vi "Load Instrument Classes_New.vi"(8 "error in (no error)":errorcluster, 11 "C.E.":refnum<class "Control Experiment.lvclass">) -> (0 "error out":errorcluster, 3 "Control Experiment":refnum<class "Control Experiment.lvclass">)   [LabVIEW 2019, in "Control Experiment.lvclass"]
uses:
  Control Experiment.lvclass
  <userlib>/LevyLab/Instrument Framework/SMOs/Instrument/Instrument.lvclass
  Control Experiment.lvclass/Control Experiment.ctl
  <userlib>/LevyLab/Lockin-Multichannel/Instrument.Lockin/Instrument.Lockin.lvclass
  C:/Program Files (x86)/National Instruments/LabVIEW 2019/user.lib/LevyLab/Instrument Framework/SMOs/Instrument/Instrument.lvclass
  Typedefs/Instrument Types--combo.ctl
  <userlib>/LevyLab/Instrument Framework/SMOs/Instrument/Instrument.lvclass/Instrument.ctl
  <userlib>/LevyLab/Krohn Hite 7008/Instrument.KH7008.lvclass
  <vilib>/Utility/Data Type/NI_Data Type.lvlib
panel:
  out "String":string
  in  "Lockin":cluster{"Lockin Address":string} caption="Instruments"
  in  "Instruments (addresses)":T1 caption="Instruments"
  in  "KH Addresses":refnum<visa-resource-name>[](array[refnum])=["COM20", "COM14"] caption="Krohn Hite"
  in  "OK":bool
  in  "Instruments (classes)":T2 {"Capacitance Bridge" items=["", "AH2500A"]; "Level" items=["", "Instrument.TC.CF", "Instrument.TC.MNK", "Instrument.Oxford1820", "instrument.PPMS", "instrument.PPMS1", "instrument.PPMS2", "instrument.PPMS3"]; "Rotator" items=["", "Instrument.TC.CF", "Instrument.TC.MNK", "Instrument.Oxford1820", "instrument.PPMS", "instrument.PPMS1", "instrument.PPMS2", "instrument.PPMS3"]; "Magnet" items=["", "Instrument.TC.CF", "Instrument.TC.MNK", "Instrument.Oxford1820", "instrument.PPMS", "instrument.PPMS1", "instrument.PPMS2", "instrument.PPMS3"]; "Temperature" items=["", "Instrument.TC.CF", "Instrument.TC.MNK", "Instrument.Oxford1820", "instrument.PPMS", "instrument.PPMS1", "instrument.PPMS2", "instrument.PPMS3"]}
  # "1. Choose or confirm instrument classes"
  # "2. Choose or confirm addresses"
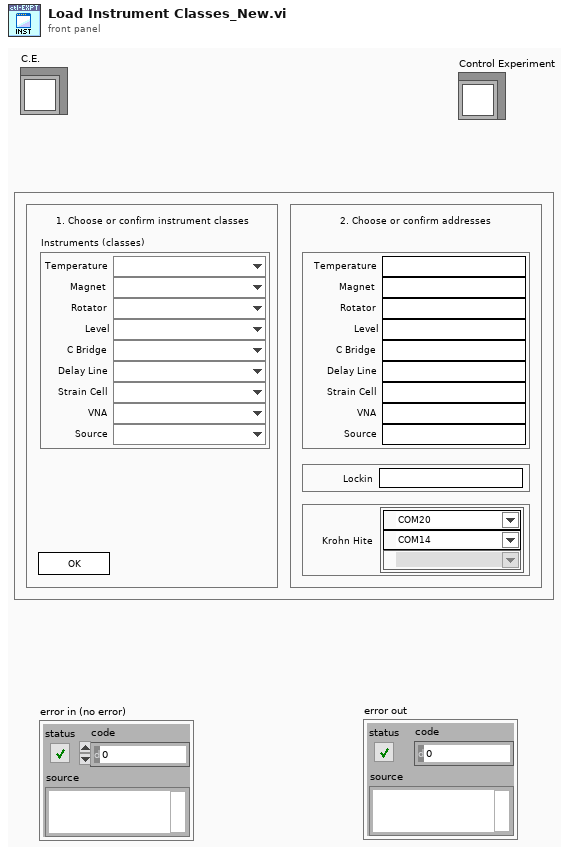
[diagram p1: front panel]
types:
  T1 = cluster{"Temperature":string, "Magnet":string, "Rotator":string, "Level":string, "Capacitance Bridge":string, "Delay Line":string, "Strain Cell":string, "VNA":string, "Source":string}
  T2 = cluster{"Temperature":u16, "Magnet":u16, "Rotator":u16, "Level":u16, "Capacitance Bridge":u16, "Delay Line":u16, "Strain Cell":u16, "VNA":u16, "Source":u16}
  T3 = enum32{"Invalid", "Standard", "Closed", "Hidden", "Minimized", "Maximized"}
  T4 = enum32{"invalid app kind", "Development System", "Run Time System", "Student Edition", "Embedded LabVIEW", "Evaluation", "Custom"}
  T5 = typedef "Control Experiment.lvclass/Instrument Types--combo.ctl" = string
  T6 = cluster{"Core":cluster{"Current VI Reference":refnum<vi>, "Close Panel on Exit?":bool}, "C.E.":refnum<class "Control Experiment.lvclass">, "Instruments":refnum<vi>, "Addresses":refnum<vi>, "Rings":refnum<vi>[], "Installed Instruments":refnum<class "Instrument.lvclass">[], "Cast Instruments":refnum<class "Instrument.lvclass">[]}
  T7 = cluster{"Current VI Reference":refnum<vi>, "Close Panel on Exit?":bool}
  T8 = enum32{"Bad", "Idle", "Run top level", "Running"}
  T9 = cluster{"class path":path, "Address":string, "Type":T5}[]
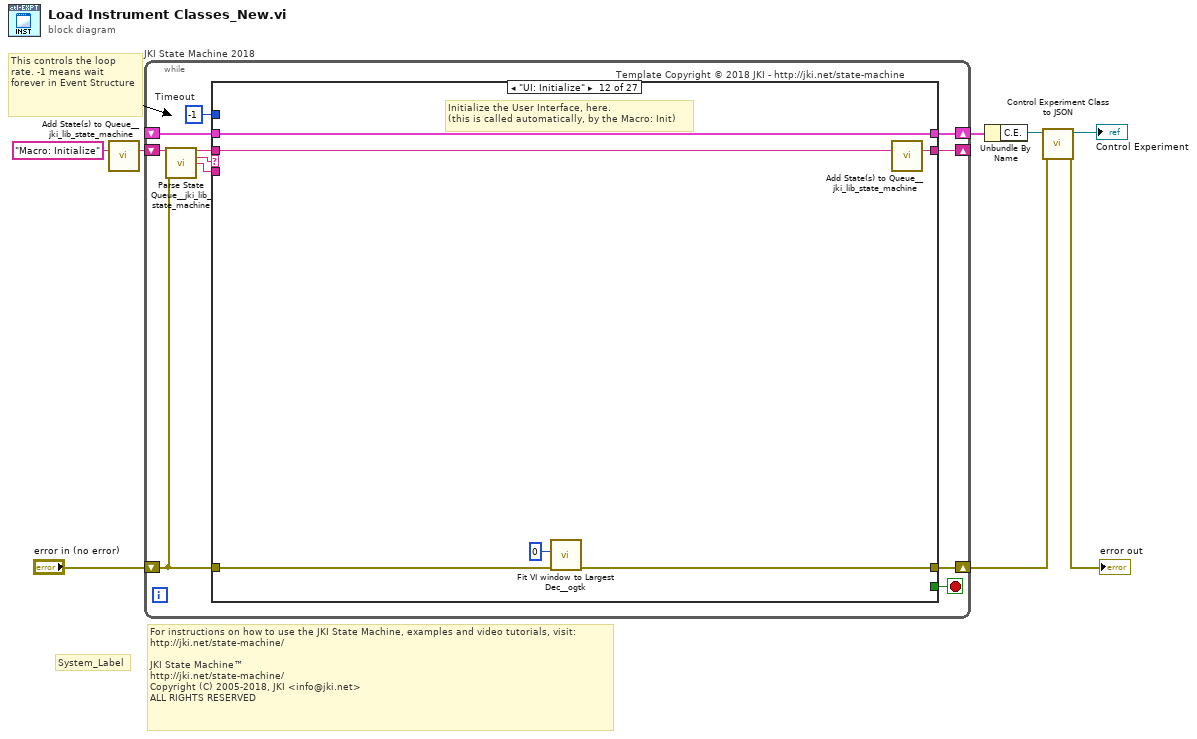
[diagram p0: block diagram]
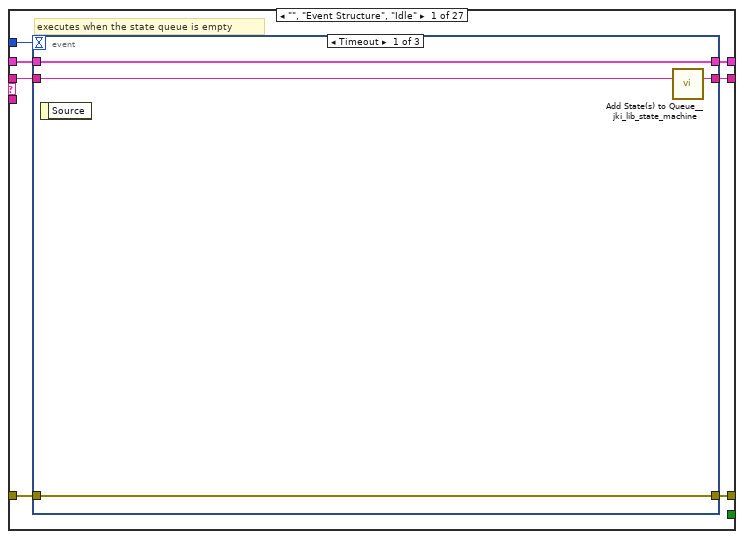
[diagram p2: hidden frame]
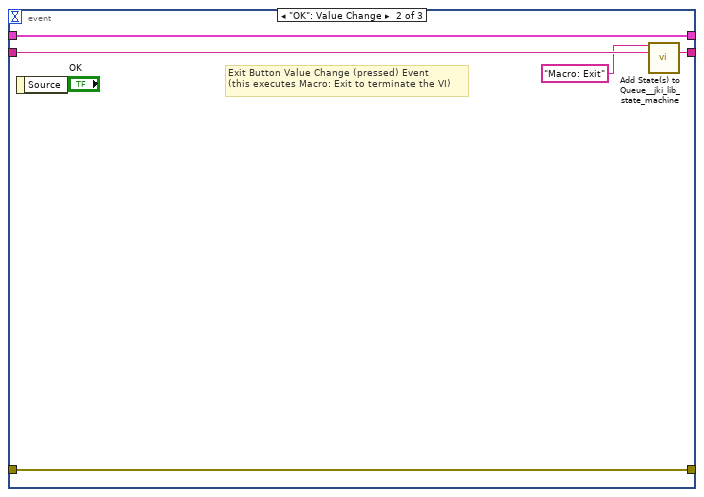
[diagram p3: hidden frame]
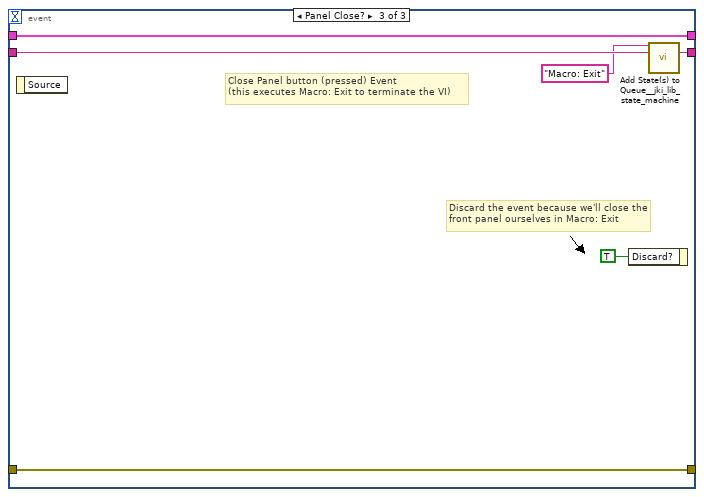
[diagram p4: hidden frame]
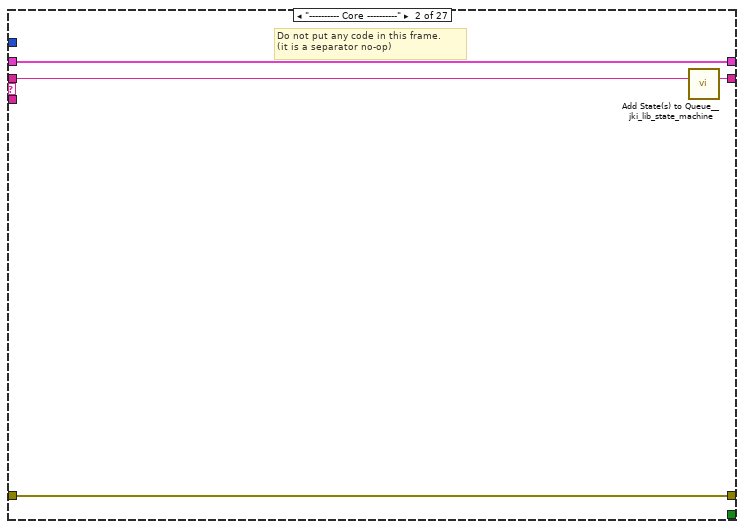
[diagram p5: hidden frame]
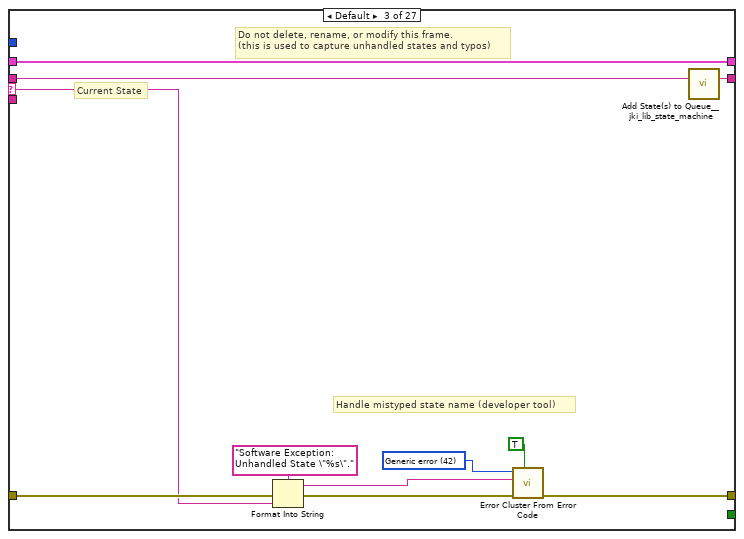
[diagram p6: hidden frame]
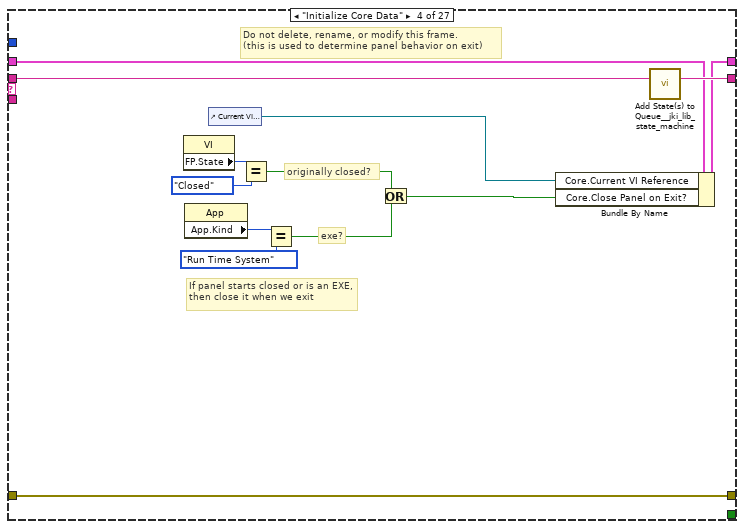
[diagram p7: hidden frame]
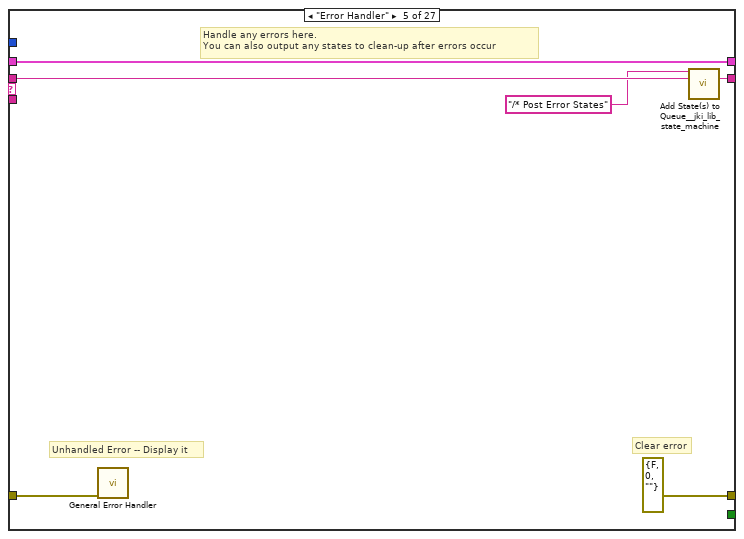
[diagram p8: hidden frame]
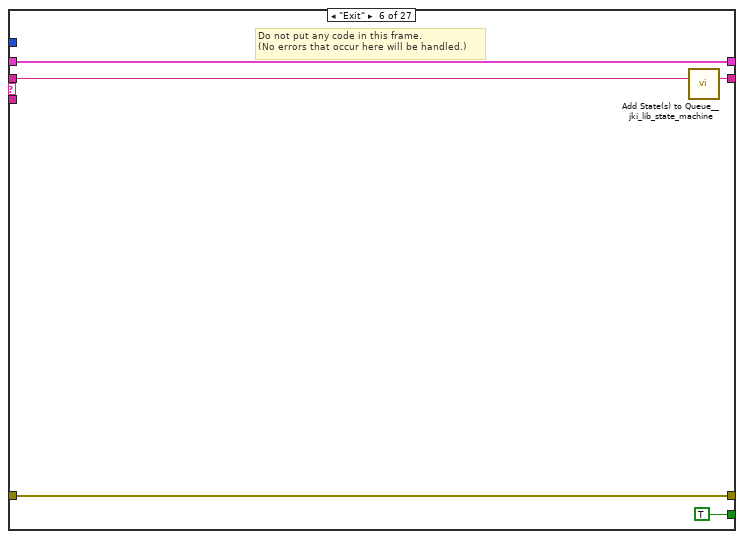
[diagram p9: hidden frame]
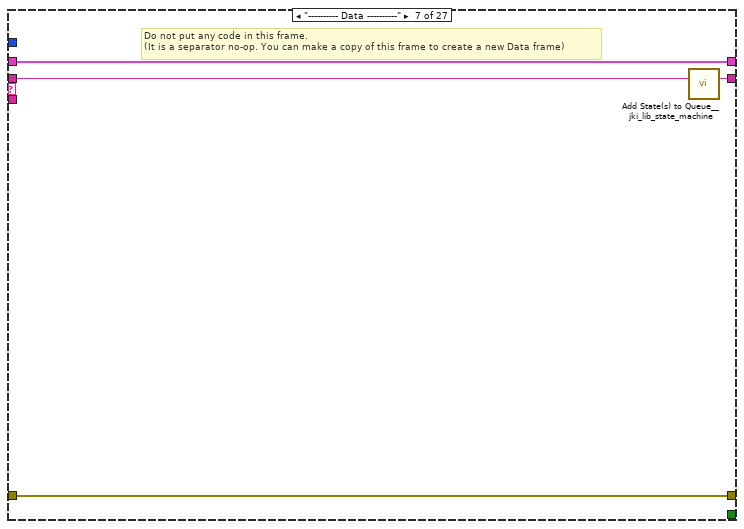
[diagram p10: hidden frame]
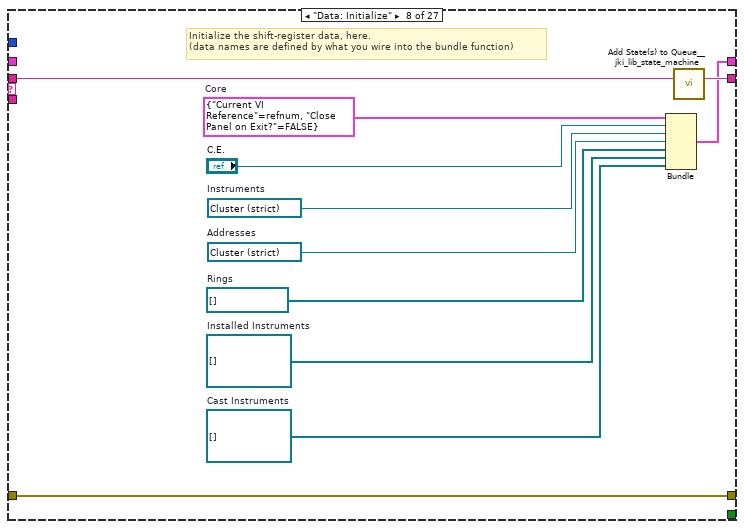
[diagram p11: hidden frame]
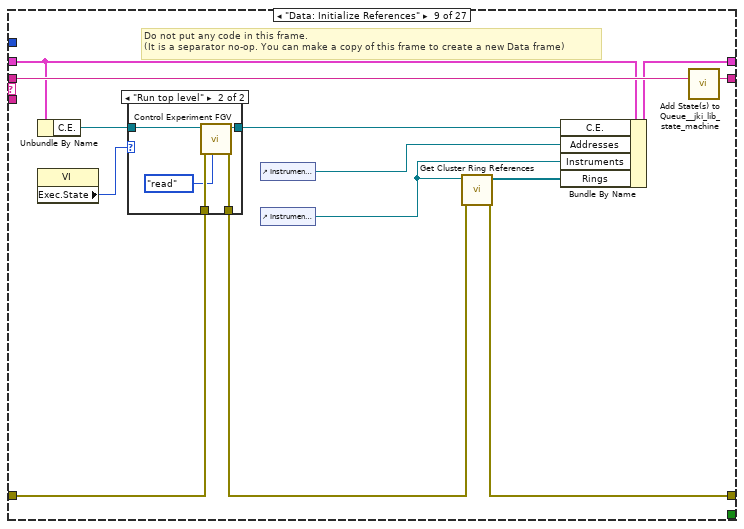
[diagram p12: hidden frame]
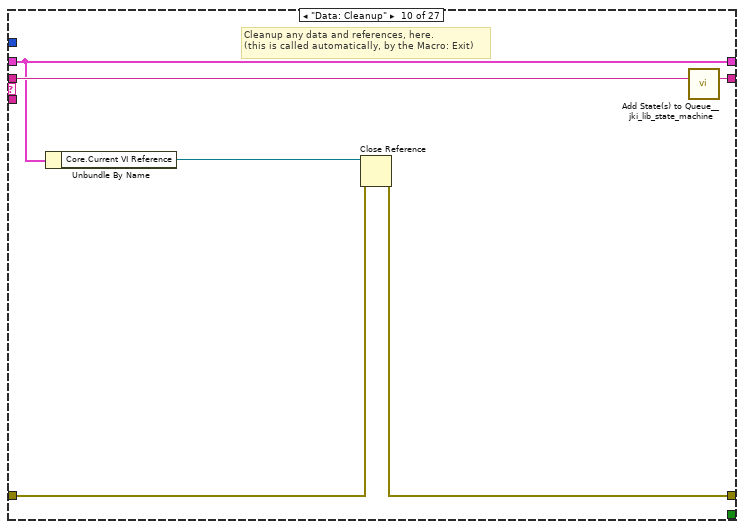
[diagram p14: hidden frame]
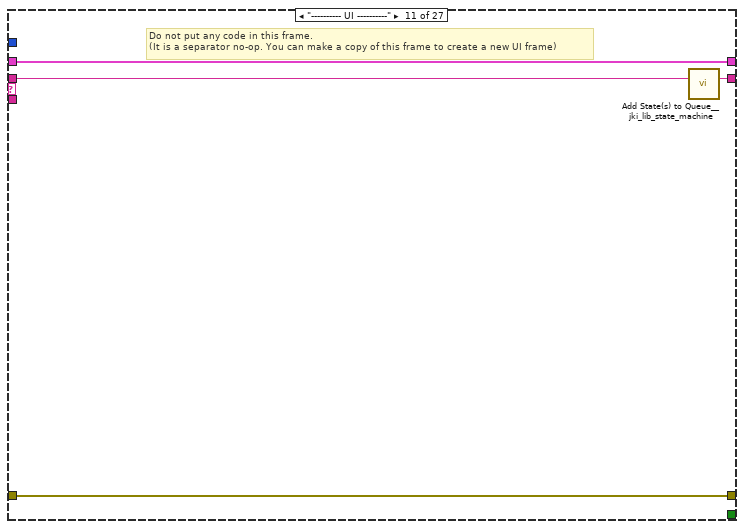
[diagram p15: hidden frame]
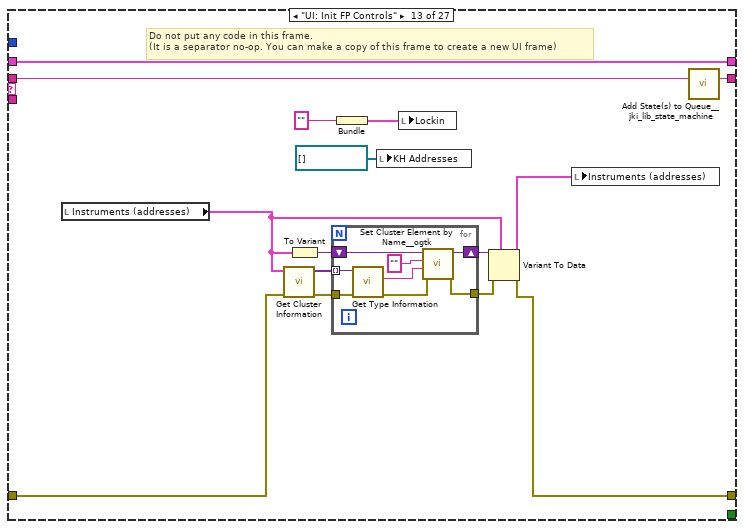
[diagram p16: hidden frame]
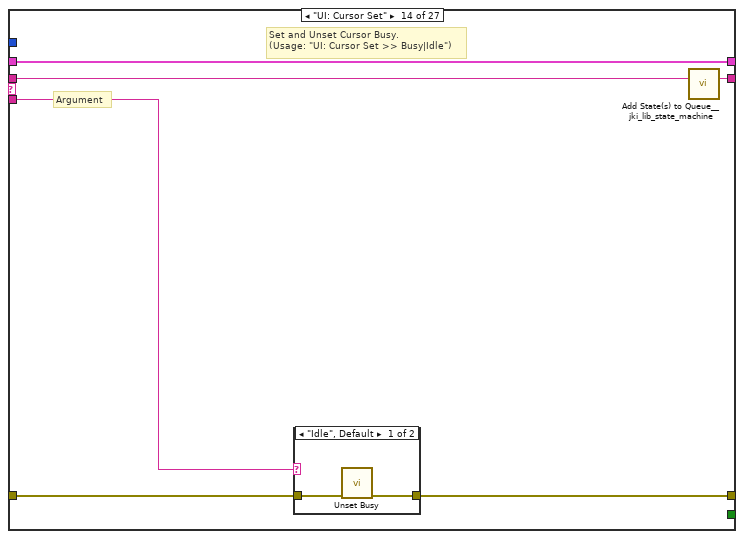
[diagram p17: hidden frame]
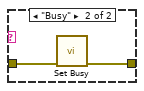
[diagram p18: hidden frame]
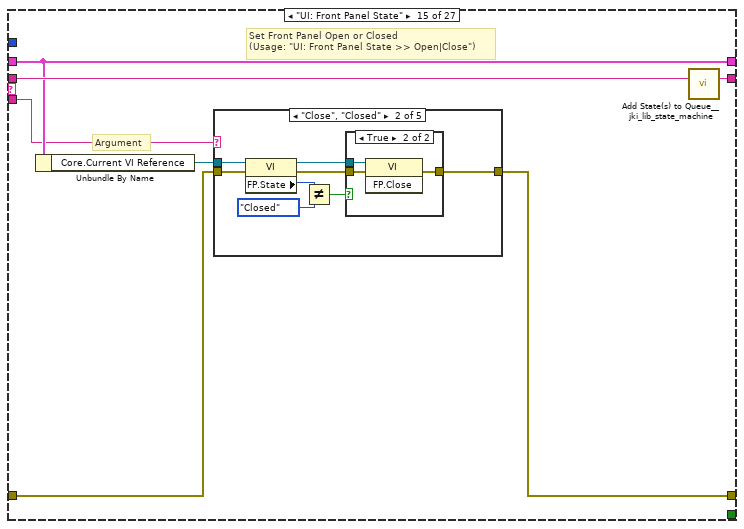
[diagram p19: hidden frame]
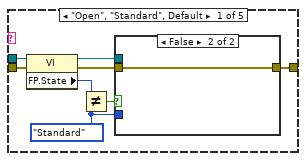
[diagram p20: hidden frame]
diagram:
  # "For instructions on how to use the JKI State Machine, examples and video tutorials, visit:\nhttp://jki.net/state-machine/\n\nJKI State Machine™\nhttp://jki.net/state-machine/\nCopyright (C) 2005-2018, JKI <info@jki.net>\nALL RIGHTS RESERVED"
  # "This controls the loop rate. -1 means wait forever in Event Structure"
  # "System_Label"
  n1 = call <vilib>:"Add State(s) to Queue__jki_lib_state_machine.vi"("State(s) in (\"\")"="Macro: Initialize") -> ("States Out"=w8:string)  [unwired: 14 in]
  n2 = while "JKI State Machine 2018" {
    shift-right: [w12] -> w6
    shift-left: _ -> [w11]
    shift-right: [w15] -> w2
    shift-left: "error in (no error)" -> [w9]
    shift-right: [w14] -> _
    shift-left: w8 -> [w16]
    stop <- w13 stop-if-true
    w10 = -1  # Timeout
    # "Template Copyright © 2018 JKI - http://jki.net/state-machine"
    n3 = call <vilib>:"Parse State Queue__jki_lib_state_machine.vi"("State Queue"=w16, "Error In (no error)"=w9) -> ("Remaining States"=w18:string, "Current State"=w19:string, "Arguments"=w17:string)  [unwired: 11 in]
    n4 = case shown="\"UI: Initialize\"" w19 {
      selector: w19 -> [_ _ w46 _ _ _ _ _ _ _ _ _ _ _ _ _ _ _ _ _ _ _ _ _ _ _ _]
      tunnel: w18 -> [w26 w45 w50 w69 w75 w80 w84 w95 w108 w121 w125 w131 w146 w160 w171 w240 w245 w256 w260 w266 w279 w299 w305 w329 w344 w363 w386]
      tunnel: w17 -> [_ _ _ _ _ _ _ _ _ _ _ _ _ w155 w165 _ _ _ _ _ _ _ _ _ _ _ _]
      tunnel: w11 -> [w24 w42 w48 w62 w72 w78 w81 _ w99 w116 w122 w127 w138 w158 w167 w237 w242 w253 w257 w263 w270 w297 w302 w326 w341 w359 w375]
      tunnel: [w23 w43 w52 w66 errorcluster {"status"=FALSE, "code"=0, "source"=""} ("error out") w77 w82 w92 w103 w117 w123 w129 w134 w156 w168 w238 w243 w254 w258 w262 w269 w296 w303 w327 w340 w356 w378] -> w15
      tunnel: w9 -> [w22 w43 w51 w66 w71 w77 w82 w92 w101 w118 w123 w128 w133 w157 w169 w238 w243 w254 w258 w261 w269 w295 w303 w327 w337 w351 w377]
      tunnel: [w25 w44 w49 w68 w74 w79 w83 w94 w107 w120 w124 w130 w145 w159 w170 w239 w244 w255 w259 w265 w278 w298 w304 w328 w343 w362 w385] -> w14
      tunnel: [_ _ _ _ _ TRUE _ _ _ _ _ _ _ _ _ _ _ _ _ _ _ _ _ _ _ _ _] -> w13
      tunnel: [w21 w42 w48 w67 w72 w78 w81 w93 w106 w116 w122 w127 w138 w158 w167 w237 w242 w253 w257 w263 w271 w297 w302 w326 w342 w360 w376] -> w12
      tunnel: w10 -> [w20 _ _ _ _ _ _ _ _ _ _ _ _ _ _ _ _ _ _ _ _ _ _ _ _ _ _]
      frame "", "Event Structure", "Idle" {
        # "executes when the state queue is empty"
        n5 = event shown="[0] Timeout" {
          selector: _ -> [_ _ _]
          dyn-events: _ -> [_ _ _]
          timeout: w20 -> [_ _ _]
          tunnel: w26 -> [w30 w35 w41]
          tunnel: [w29 w34 w40] -> w25
          tunnel: w24 -> [w27 w32 w38]
          tunnel: [w28 w33 w39] -> w23
          tunnel: w22 -> [w28 w33 w39]
          tunnel: [w27 w32 w38] -> w21
          event Timeout {
            n6 = event-data() -> ()  [unwired: 1 in, 1 out]
            n7 = call <vilib>:"Add State(s) to Queue__jki_lib_state_machine.vi"("State(s) in (\"\")"=w30) -> ("States Out"=w29:string)  [unwired: 14 in]
          }
          event "OK": Value Change {
            # "Exit Button Value Change (pressed) Event\n(this executes Macro: Exit to terminate the VI)"
            n8 = event-data() -> ()  [unwired: 1 in, 1 out]
            n9 = call <vilib>:"Add State(s) to Queue__jki_lib_state_machine.vi"("State(s) in Front (\"\")"="Macro: Exit", "State(s) in (\"\")"=w35) -> ("States Out"=w34:string)  [unwired: 13 in]
          }
          event Panel Close? {
            # "Discard the event because we'll close the front panel ourselves in Macro: Exit"
            # "Close Panel button (pressed) Event\n(this executes Macro: Exit to terminate the VI)"
            n10 = event-data() -> ()  [unwired: 1 in, 1 out]
            n11 = event-data("Discard?"=TRUE) -> ()  [unwired: 1 in, 1 out]
            n12 = call <vilib>:"Add State(s) to Queue__jki_lib_state_machine.vi"("State(s) in Front (\"\")"="Macro: Exit", "State(s) in (\"\")"=w41) -> ("States Out"=w40:string)  [unwired: 13 in]
          }
        }
      }
      frame "---------- Core ----------" {
        # "Do not put any code in this frame.\n(it is a separator no-op)"
        n13 = call <vilib>:"Add State(s) to Queue__jki_lib_state_machine.vi"("State(s) in (\"\")"=w45) -> ("States Out"=w44:string)  [unwired: 14 in]
      }
      frame Default {
        w55 = 42 items=["No error", "Argument error", "Memory is full", "Out of zone", "End of file", "File already open", "Generic file I/O error", "File not found", "File permission error", "Disk is full", "Duplicate path", "Too many files open", "System feature not enabled", "Resource file not found", "Cannot add resource", "Resource not found", "Image not found", "Image memory error", "Pen does not exist", "Config type invalid", "Config token not found", "Config parse error", "Config memory error", "Bad external code format", "Bad external code offset", "External code not present", "Null window", "Destroy window error", "Null menu", "Print aborted", "Bad print record", "Print driver error", "Windows error during printing", "Memory error during printing", "Print dialog error", "Generic print error", "Invalid device refnum", "Device not found", "Device parameter error", "Device unit error", "Cannot open device", "Device call aborted", "Generic error", "Cancelled by user", "Object ID too low", "Object ID too high", "Object not in heap", "Unknown heap", "Unknown object (invalid DefProc)", "Unknown object (DefProc not in table)", "Message out of range", "Invalid (null) method", "Unknown message", "Manager call not supported", "Bad address", "Network operation in progress", "Network operation timed out", "Connection is busy", "Network attribute not supported", "Network error", "Address in use", "System out of memory", "Connection aborted", "Connection refused", "Not connected", "Already connected", "Connection closed", "Initialization error (interapplication manager)", "Bad occurrence", "Wait on unbound occurrence handler", "Occurrence queue overflow", "Datalog type conflict", "Unused", "Unrecognized type (interapplication manager)", "Memory corrupt", "Failed to make temporary DLL", "Old CIN version", "Drag socket not found", "Failed to load drop-object", "Failed to register OLE object", "Failed to release OLE object", "Format specifier type mismatch", "Unknown format specifier", "Too few format specifiers", "Too many format specifiers", "Scan failed", "Newer CIN version", "Error converting to variant", "Runtime menu error", "Password tampered", "Variant attribute not found", "Incompatible variant data type", "Event data is not available", "Event Store is not present", "Occurrence is not found", "Event Queue is not created", "Event info is not available", "Refnum passed is NULL", "Error retrieving Class GUID", "Error retrieving CoClass GUID", "Error retrieving TypeLib GUID.", "Bad built application magic bytes.", "Specific driver is different from the specific driver associated with the Logical Name.", "There is no session opened to the class driver.", "Max Error", "MAX - Error with config objects", "MAX - Error loading configuration", "MAX - Group not supported"]
        # "Current State"
        # "Do not delete, rename, or modify this frame.\n(this is used to capture unhandled states and typos)"
        # "Handle mistyped state name (developer tool)"
        n14 = Format Into String(format string="Software Exception: Unhandled State \"%s\"." ("message"), error in=w51, w46) -> (resulting string=w54:string, error out=w53:errorcluster)  [unwired: 1 in]
        n15 = call <vilib>:"Error Cluster From Error Code.vi"("show call chain? (False)"=TRUE, "error in (no error)"=w53, "error message (\"\")"=w54, "error code (0)"=w55) -> ("error out"=w52:errorcluster)  [unwired: 5 in]
        n16 = call <vilib>:"Add State(s) to Queue__jki_lib_state_machine.vi"("State(s) in (\"\")"=w50) -> ("States Out"=w49:string)  [unwired: 14 in]
      }
      frame "Initialize Core Data" {
        # "Do not delete, rename, or modify this frame.\n(this is used to determine panel behavior on exit)"
        # "originally closed?"
        # "exe?"
        # "If panel starts closed or is an EXE, then close it when we exit"
        n17 = property class="VI"() -> ("FP.State"=w59:T3)  [unwired: 2 in, 2 out]
        n18 = property class="App"() -> ("App.Kind"=w65:T4)  [unwired: 2 in, 2 out]
        n19 = control-ref of="Current VI Reference"() -> (w60:refnum<vi>)
        n20 = Equal?(x=w59, y=T3."Closed" ("Front Panel Window:State")) -> (x = y?=w57:bool)
        n21 = Equal?(x=w65, y=T4."Run Time System" ("Application:Kind")) -> (x = y?=w63:bool)
        n22 = Or(x=w57, y=w63) -> (x .or. y?=w61:bool)
        n23 = Bundle By Name(cluster=w62, "Core.Current VI Reference"=w60, "Core.Close Panel on Exit?"=w61) -> (w67:T6)
        n24 = call <vilib>:"Add State(s) to Queue__jki_lib_state_machine.vi"("State(s) in (\"\")"=w69) -> ("States Out"=w68:string)  [unwired: 14 in]
      }
      frame "Error Handler" {
        # "Unhandled Error -- Display it"
        # "Handle any errors here.\nYou can also output any states to clean-up after errors occur"
        # "Clear error"
        n25 = call <vilib>:"General Error Handler.vi"("error in (no error)"=w71) -> ()  [unwired: 10 in, 5 out]
        n26 = call <vilib>:"Add State(s) to Queue__jki_lib_state_machine.vi"("State(s) in Front (\"\")"="/* Post Error States", "State(s) in (\"\")"=w75) -> ("States Out"=w74:string)  [unwired: 13 in]
      }
      frame "Exit" {
        # "Do not put any code in this frame.\n(No errors that occur here will be handled.)"
        n27 = call <vilib>:"Add State(s) to Queue__jki_lib_state_machine.vi"("State(s) in (\"\")"=w80) -> ("States Out"=w79:string)  [unwired: 14 in]
      }
      frame "---------- Data ----------" {
        # "Do not put any code in this frame.\n(It is a separator no-op. You can make a copy of this frame to create a new Data frame)"
        n28 = call <vilib>:"Add State(s) to Queue__jki_lib_state_machine.vi"("State(s) in (\"\")"=w84) -> ("States Out"=w83:string)  [unwired: 14 in]
      }
      frame "Data: Initialize" {
        w85 = refnum<vi> refnum  # Addresses
        w87 = refnum<vi> refnum  # Instruments
        w88 = refnum<class "Instrument.lvclass">[] []  # Cast Instruments
        w89 = refnum<vi>[] []  # Rings
        w90 = refnum<class "Instrument.lvclass">[] []  # Installed Instruments
        w91 = T7 {"Current VI Reference"=refnum, "Close Panel on Exit?"=FALSE}  # Core
        # "Initialize the shift-register data, here.\n(data names are defined by what you wire into the bundle function)"
        n29 = Bundle("Core"=w91, "C.E."="C.E.", "Instruments"=w87, "Addresses"=w85, "Rings"=w89, "Installed Instruments"=w90, "Cast Instruments"=w88) -> (w93:T6)  [unwired: 1 in]
        n30 = call <vilib>:"Add State(s) to Queue__jki_lib_state_machine.vi"("State(s) in (\"\")"=w95) -> ("States Out"=w94:string)  [unwired: 14 in]
      }
      frame "Data: Initialize References" {
        # "Do not put any code in this frame.\n(It is a separator no-op. You can make a copy of this frame to create a new Data frame)"
        n31 = Unbundle By Name(w99) -> ("C.E."=w98:refnum<class "Control Experiment.lvclass">)
        n32 = property class="VI"() -> ("Exec.State"=w97:T8)  [unwired: 2 in, 2 out]
        n33 = case shown="\"Run top level\"" w97 {
          tunnel: [w109 w115] -> w102
          tunnel: w101 -> [w109 w114]
          tunnel: [w110 w112] -> w100
          tunnel: w98 -> [w110 w111]
          frame Default {
          }
          frame "Run top level" {
            n34 = call "Control Experiment FGV.vi"("Function"=enum16{"read", "write"}."read", "error in (no error)"=w114, "Control Experiment.lvclass"=w111) -> ("error out"=w115:errorcluster, "Control Experiment.lvclass out"=w112:refnum<class "Control Experiment.lvclass">)  [unwired: 7 in]
          }
        }
        n35 = control-ref of="Instruments (addresses)"() -> (w96:refnum<vi>)
        n36 = control-ref of="Instruments (classes)"() -> (w105:refnum<vi>)
        n37 = call "Get Cluster Ring References.vi"("error in (no error)"=w102, "Cluster Reference in"=w105) -> ("error out"=w103:errorcluster, "Ring References"=w104:refnum<vi>[])  [unwired: 8 in]
        n38 = Bundle By Name(cluster=w99, "C.E."=w100, "Addresses"=w96, "Instruments"=w105, "Rings"=w104) -> (w106:T6)
        n39 = call <vilib>:"Add State(s) to Queue__jki_lib_state_machine.vi"("State(s) in (\"\")"=w108) -> ("States Out"=w107:string)  [unwired: 14 in]
      }
      frame "Data: Cleanup" {
        # "Cleanup any data and references, here.\n(this is called automatically, by the Macro: Exit)"
        n40 = Unbundle By Name(w116) -> ("Core.Current VI Reference"=w119:refnum<vi>)
        n41 = Close Reference(reference=w119, error in (no error)=w118) -> (error out=w117:errorcluster)
        n42 = call <vilib>:"Add State(s) to Queue__jki_lib_state_machine.vi"("State(s) in (\"\")"=w121) -> ("States Out"=w120:string)  [unwired: 14 in]
      }
      frame "---------- UI ----------" {
        # "Do not put any code in this frame.\n(It is a separator no-op. You can make a copy of this frame to create a new UI frame)"
        n43 = call <vilib>:"Add State(s) to Queue__jki_lib_state_machine.vi"("State(s) in (\"\")"=w125) -> ("States Out"=w124:string)  [unwired: 14 in]
      }
      frame "UI: Initialize" {
        # "Initialize the User Interface, here.\n(this is called automatically, by the Macro: Init)"
        n44 = call <userlib>:"Fit VI window to Largest Dec__ogtk.vi"("error in (no error)"=w128, "border spacing (2 px)"=0) -> ("error out"=w129:errorcluster)  [unwired: 4 in, 1 out]
        n45 = call <vilib>:"Add State(s) to Queue__jki_lib_state_machine.vi"("State(s) in (\"\")"=w131) -> ("States Out"=w130:string)  [unwired: 14 in]
      }
      frame "UI: Init FP Controls" {
        # "Do not put any code in this frame.\n(It is a separator no-op. You can make a copy of this frame to create a new UI frame)"
        n46 = local read "Instruments (addresses)"() -> (w136:T1)
        n47 = call <vilib>:"Get Cluster Information.vi"("error in (no error)"=w133, "variant"=w136) -> ("error out"=w142:errorcluster, "cluster elements"=w144:variant[])  [unwired: 8 in]
        n48 = To Variant(anything=w136) -> (Variant=w137:variant)
        n49 = for {
          tunnel: w144 -> [w154] mode=indexing
          shift-right: [w152] -> w143
          shift-left: w137 -> [w153]
          tunnel: w142 -> [w147]
          tunnel: [w148] -> w141
          n50 = call <vilib>:"Get Type Information.vi"("error in (no error)"=w147, "variant"=w154) -> ("error out"=w149:errorcluster, "name"=w150:string)  [unwired: 5 in, 3 out]
          n51 = call <userlib>:"Set Cluster Element by Name__ogtk.vi"("error in (no error)"=w149, "Element Name (\"\": New Element Data Name)"=w150, "New Element Value"="", "Cluster"=w153) -> ("error out"=w148:errorcluster, "VCluster out"=w152:variant)  [unwired: 5 in, 1 out]
        }
        n52 = Bundle("Lockin Address"="") -> (w132:cluster{"Lockin Address":string})  [unwired: 1 in]
        n53 = local write "KH Addresses"(refnum<visa-resource-name>[] [] ("KH Addresses")) -> ()
        n54 = local write "Lockin"(w132) -> ()
        n55 = Variant To Data(error in=w141, type=w136, Variant=w143) -> (data=w135:T1, error out=w134:errorcluster)
        n56 = local write "Instruments (addresses)"(w135) -> ()
        n57 = call <vilib>:"Add State(s) to Queue__jki_lib_state_machine.vi"("State(s) in (\"\")"=w146) -> ("States Out"=w145:string)  [unwired: 14 in]
      }
      frame "UI: Cursor Set" {
        # "Argument"
        # "Set and Unset Cursor Busy.\n(Usage: \"UI: Cursor Set >> Busy|Idle\")"
        n58 = case shown="\"Idle\", Default" w155 {
          tunnel: w157 -> [w162 w164]
          tunnel: [w161 w163] -> w156
          frame "Idle", Default {
            n59 = call <vilib>:"Unset Busy.vi"("error in (no error)"=w162) -> ("error out"=w161:errorcluster)  [unwired: 10 in]
          }
          frame "Busy" {
            n60 = call <vilib>:"Set Busy.vi"("error in (no error)"=w164) -> ("error out"=w163:errorcluster)  [unwired: 9 in, 1 out]
          }
        }
        n61 = call <vilib>:"Add State(s) to Queue__jki_lib_state_machine.vi"("State(s) in (\"\")"=w160) -> ("States Out"=w159:string)  [unwired: 14 in]
      }
      frame "UI: Front Panel State" {
        # "Argument"
        # "Set Front Panel Open or Closed\n(Usage: \"UI: Front Panel State >> Open|Close\")"
        n62 = Unbundle By Name(w167) -> ("Core.Current VI Reference"=w166:refnum<vi>)
        n63 = case shown="\"Close\", \"Closed\"" w165 {
          tunnel: w169 -> [w177 w192 w203 w216 w229]
          tunnel: [w179 w193 w205 w218 w231] -> w168
          tunnel: w166 -> [w178 w190 w204 w217 w230]
          frame "Open", "Standard", Default {
            w172 = T3."Standard" ("State")
            n64 = property class="VI"(reference=w178, error in=w177) -> (reference out=w175:refnum<vi>, error out=w176:errorcluster, "FP.State"=w174:T3)
            n65 = Not Equal?(x=w174, y=w172) -> (x != y?=w173:bool)
            n66 = case shown="False" w173 {
              tunnel: [w183 w185] -> w179
              tunnel: w176 -> [w182 w185]
              tunnel: w175 -> [w181 _]
              tunnel: w172 -> [w180 _]
              frame True {
                n67 = invoke class="VI" method="FP.Open"(reference=w181, error in=w182, "Activate"=TRUE, "State"=w180) -> (error out=w183:errorcluster)  [unwired: 1 in, 4 out]
              }
              frame False {
              }
            }
          }
          frame "Close", "Closed" {
            n68 = property class="VI"(reference=w190, error in=w192) -> (reference out=w189:refnum<vi>, error out=w191:errorcluster, "FP.State"=w187:T3)
            n69 = Not Equal?(x=w187, y=T3."Closed" ("Front Panel Window:State")) -> (x != y?=w186:bool)
            n70 = case shown="True" w186 {
              tunnel: [w194 w197] -> w193
              tunnel: w191 -> [w194 w196]
              tunnel: w189 -> [_ w195]
              frame False {
              }
              frame True {
                n71 = invoke class="VI" method="FP.Close"(reference=w195, error in=w196) -> (error out=w197:errorcluster)  [unwired: 1 in, 2 out]
              }
            }
          }
          frame "Hidden", "Hide" {
            w198 = T3."Hidden" ("State")
            n72 = property class="VI"(reference=w204, error in=w203) -> (reference out=w201:refnum<vi>, error out=w202:errorcluster, "FP.State"=w200:T3)
            n73 = Not Equal?(x=w200, y=w198) -> (x != y?=w199:bool)
            n74 = case shown="True" w199 {
              tunnel: [w209 w210] -> w205
              tunnel: w202 -> [w208 w210]
              tunnel: w201 -> [w207 _]
              tunnel: w198 -> [w206 _]
              frame True {
                n75 = invoke class="VI" method="FP.Open"(reference=w207, error in=w208, "State"=w206) -> (error out=w209:errorcluster)  [unwired: 2 in, 4 out]
              }
              frame False {
              }
            }
          }
          frame "Minimize", "Minimized" {
            w211 = T3."Minimized" ("State")
            n76 = property class="VI"(reference=w217, error in=w216) -> (reference out=w214:refnum<vi>, error out=w215:errorcluster, "FP.State"=w213:T3)
            n77 = Not Equal?(x=w213, y=w211) -> (x != y?=w212:bool)
            n78 = case shown="True" w212 {
              tunnel: [w222 w223] -> w218
              tunnel: w215 -> [w221 w223]
              tunnel: w214 -> [w220 _]
              tunnel: w211 -> [w219 _]
              frame True {
                n79 = invoke class="VI" method="FP.Open"(reference=w220, error in=w221, "State"=w219) -> (error out=w222:errorcluster)  [unwired: 2 in, 4 out]
              }
              frame False {
              }
            }
          }
          frame "Maximize", "Maximized" {
            w224 = T3."Maximized" ("State")
            n80 = property class="VI"(reference=w230, error in=w229) -> (reference out=w227:refnum<vi>, error out=w228:errorcluster, "FP.State"=w226:T3)
            n81 = Not Equal?(x=w226, y=w224) -> (x != y?=w225:bool)
            n82 = case shown="True" w225 {
              tunnel: [w235 w236] -> w231
              tunnel: w228 -> [w234 w236]
              tunnel: w227 -> [w233 _]
              tunnel: w224 -> [w232 _]
              frame True {
                n83 = invoke class="VI" method="FP.Open"(reference=w233, error in=w234, "State"=w232) -> (error out=w235:errorcluster)  [unwired: 2 in, 4 out]
              }
              frame False {
              }
            }
          }
        }
        n84 = call <vilib>:"Add State(s) to Queue__jki_lib_state_machine.vi"("State(s) in (\"\")"=w171) -> ("States Out"=w170:string)  [unwired: 14 in]
      }
      frame "---------- Macro ----------" {
        # "Do not put any code in this frame.\n(It is a separator no-op. You can make a copy of this frame to create a new Macro frame)"
        n85 = call <vilib>:"Add State(s) to Queue__jki_lib_state_machine.vi"("State(s) in (\"\")"=w240) -> ("States Out"=w239:string)  [unwired: 14 in]
      }
      frame "Macro: Initialize" {
        # "Initialization Macro\n(This is called once, when the VI starts)"
        n86 = call <vilib>:"Add State(s) to Queue__jki_lib_state_machine.vi"("State(s) in Front (\"\")"="Data: Initialize\nInitialize Core Data\nUI: Initialize\nUI: Front Panel State >> Open\n\nData: Initialize References\nUI: Init FP Controls\n\nRings: Empty Rings\nRings: List Installed\nRings: Installed to Rings\n\nRings: Init Addresses", "State(s) in (\"\")"=w245) -> ("States Out"=w244:string)  [unwired: 13 in]
      }
      frame "Macro: Exit" {
        # "Exit Macro\n(This is called once, when the VI exits)"
        n87 = Unbundle By Name(w253) -> ("Core.Close Panel on Exit?"=w252:bool)
        n88 = Select(t="UI: Front Panel State >> Close", s=w252, f="") -> (s? t:f=w249:string)
        n89 = call <vilib>:"Add State(s) to Queue__jki_lib_state_machine.vi"("State(s) in Front (\"\")"="Instruments: Init Lockin\nInstruments: Init KH\nInstruments: Init Instruments" ("State(s) in Front (\"\")"), "State(s) in (\"\")"=w249, "State(s) at Back (\"\")"="Data: Cleanup\nExit") -> ("States Out"=w247:string)  [unwired: 12 in]
        n90 = call <vilib>:"Add State(s) to Queue__jki_lib_state_machine.vi"("State(s) in Front (\"\")"=w247, "State(s) in (\"\")"=w256) -> ("States Out"=w255:string)  [unwired: 13 in]
      }
      frame "---------- Rings ----------" {
        # "Template Separator\n(You can make a copy of, or modify, this frame)"
        n91 = call <vilib>:"Add State(s) to Queue__jki_lib_state_machine.vi"("State(s) in (\"\")"=w260) -> ("States Out"=w259:string)  [unwired: 14 in]
      }
      frame "Rings: Empty Rings" {
        # "Template Separator\n(You can make a copy of, or modify, this frame)"
        n92 = Unbundle By Name(w263) -> ("Rings"=w264:refnum<vi>[])
        n93 = call "Empty Rings.vi"("error in (no error)"=w261, "Ring References"=w264) -> ("error out"=w262:errorcluster)  [unwired: 8 in, 1 out]
        n94 = call <vilib>:"Add State(s) to Queue__jki_lib_state_machine.vi"("State(s) in (\"\")"=w266) -> ("States Out"=w265:string)  [unwired: 14 in]
      }
      frame "Rings: List Installed" {
        # "List all classes in \\user.lib\\LevyLab\n(but not \\user.lib\\LevyLab\\Instrument Framework\\\nor Build Support\\)"
        # "Your code here.\n(You can make a copy of, or modify, this frame)"
        n95 = call <userlib>:"User Library__ogtk.vi"() -> ("User Library (+ Relative)"=w277:path)  [unwired: 1 in]
        n96 = Build Path(base path=w277, name or relative path="LevyLab") -> (appended path=w275:path)
        n97 = call <vilib>:"Recursive File List.vi"("Folders to Exclude"=string[] ["Instrument Framework", "Build Support"], "pattern"="*.lvclass", "Folder Path"=w275) -> ("All Files in Dir"=w276:path[])  [unwired: 4 in, 4 out]
        n98 = for {
          tunnel: w276 -> [w282] mode=indexing
          tunnel: [w287] -> w268 mode=indexing if=w285
          tunnel: w269 -> [w284]
          tunnel: ["" ("String 2")] -> w267
          # "Find children of Instrument"
          n99 = call <vilib>:"Get LV Class Default Value.vi"("error in (no error)"=w284, "class path"=w282) -> ("error out"=w290:errorcluster, "object"=w291:refnum<class>)  [unwired: 8 in]
          n100 = To More Specific Class(target class=refnum<class "Instrument.lvclass"> refnum ("Instrument"), reference=w291, error in=w290) -> (specific class reference=w287:refnum<class "Instrument.lvclass">, error out=w289:errorcluster)
          n101 = Format Into String(format string="Loading...\n %s", w282) -> (resulting string=→"String":string)  [unwired: 2 in, 1 out]
          n102 = Unbundle By Name(w289) -> ("status"=w288:bool)
          n103 = Not(x=w288) -> (.not. x?=w285:bool)
        }
        n104 = Bundle By Name(cluster=w270, "Installed Instruments"=w268) -> (w271:T6)
        n105 = local write "String"(w267) -> ()
        n106 = call <vilib>:"Add State(s) to Queue__jki_lib_state_machine.vi"("State(s) in (\"\")"=w279) -> ("States Out"=w278:string)  [unwired: 14 in]
      }
      frame "Rings: Installed to Rings" {
        # "Your code here.\n(You can make a copy of, or modify, this frame)"
        n107 = Unbundle By Name(w297) -> ("C.E."=w294:refnum<class "Control Experiment.lvclass">, "Rings"=w292:refnum<vi>[], "Installed Instruments"=w293:refnum<class "Instrument.lvclass">[])
        n108 = call "Installed Classes to Rings.vi"("error in (no error)"=w295, "Installed"=w293, "Rings"=w292, "C.E."=w294) -> ("error out"=w296:errorcluster)  [unwired: 6 in, 1 out]
        n109 = call <vilib>:"Add State(s) to Queue__jki_lib_state_machine.vi"("State(s) in (\"\")"=w299) -> ("States Out"=w298:string)  [unwired: 14 in]
      }
      frame "Rings: Init Addresses" {
        # "Template Separator\n(You can make a copy of, or modify, this frame)"
        n110 = Unbundle By Name(w302) -> ("C.E."=w301:refnum<class "Control Experiment.lvclass">)  [unwired: 1 out]
        n111 = Unbundle By Name(w301) -> ("Instruments"=w300:T9)
        n112 = for {
          tunnel: w300 -> [w306] mode=indexing
          n113 = Unbundle By Name(w306) -> ("Address"=w308:string, "Type"=w307:T5)
          n114 = case shown="\"Lockin\"" w307 {
            selector: w307 -> [_ _ w321]
            tunnel: w308 -> [w309 w319 w322]
            frame "KH7008" {
              n115 = local read "KH Addresses"() -> (w310:refnum<visa-resource-name>[])
              n116 = Array Size(array=w310) -> (size(s)=w312:i32)
              n117 = case shown="Default" w312 {
                tunnel: w309 -> [w314 w317]
                tunnel: [w313 w316] -> w311
                tunnel: w310 -> [_ w315]
                frame 0 {
                  n118 = Build Array(w314) -> (w313:string[])
                }
                frame Default {
                  n119 = Build Array (concatenate)(w315, w317) -> (w316:refnum<visa-resource-name>[])
                }
              }
              n120 = local write "KH Addresses"(w311) -> ()
            }
            frame "Lockin" {
              n121 = Bundle("Address"=w319) -> (w318:cluster{"Address":string})  [unwired: 1 in]
              n122 = local write "Lockin"(w318) -> ()
            }
            frame Default {
              n123 = local read "Instruments (addresses)"() -> (w320:T1)
              n124 = call <userlib>:"Set Cluster Element by Name__ogtk.vi"("Element Name (\"\": New Element Data Name)"=w321, "New Element Value"=w322, "Cluster"=w320) -> ("error out"=w325:errorcluster, "VCluster out"=w324:variant)  [unwired: 6 in, 1 out]
              n125 = Variant To Data(error in=w325, type=w320, Variant=w324) -> (data=w323:T1)  [unwired: 1 out]
              n126 = local write "Instruments (addresses)"(w323) -> ()
            }
          }
        }
        n127 = call <vilib>:"Add State(s) to Queue__jki_lib_state_machine.vi"("State(s) in (\"\")"=w305) -> ("States Out"=w304:string)  [unwired: 14 in]
      }
      frame "---------- Instruments ----------" {
        # "Template Separator\n(You can make a copy of, or modify, this frame)"
        n128 = call <vilib>:"Add State(s) to Queue__jki_lib_state_machine.vi"("State(s) in (\"\")"=w329) -> ("States Out"=w328:string)  [unwired: 14 in]
      }
      frame "Instruments: Init Lockin" {
        # "Template Separator\n(You can make a copy of, or modify, this frame)"
        n129 = Unbundle By Name(w341) -> ("C.E."=w339:refnum<class "Control Experiment.lvclass">)
        n130 = Unbundle("Lockin") -> ("Lockin Address"=w330:string)
        n131 = call <userlib>:"Write Hardware Address.vi"("error in (no error)"=w337, "Address"=w330, "Instrument in"=refnum<class "Instrument.Lockin.lvclass"> refnum ("Instrument.Lockin in")) -> ("error out"=w334:errorcluster, "Instrument out"=w332:refnum<class "Instrument.Lockin.lvclass">)  [unwired: 7 in]
        n132 = call "Insert Instrument Class by Name.vi"("error in (no error)"=w334, "Type"=T5 "Lockin", "Instrument in"=w332, "Control Experiment in"=w339) -> ("error out"=w336:errorcluster, "Control Experiment out"=w338:refnum<class "Control Experiment.lvclass">)  [unwired: 4 in, 2 out]
        n133 = disable-structure shown="Disabled" {
          disable-tunnel: w330 -> [w347 _]
          disable-tunnel: [w346 w348] -> w340
          disable-tunnel: w337 -> [w345 _]
          disable-tunnel: w336 -> [_ w348]
          frame Disabled {
            n134 = call-dynamic "Open.vi"("error in (no error)"=w345, "address"=w347) -> ("error out"=w346:errorcluster)  [unwired: 8 in, 1 out]
          }
          frame Enabled {
          }
        }
        n135 = Bundle By Name(cluster=w341, "C.E."=w338) -> (w342:T6)
        n136 = call <vilib>:"Add State(s) to Queue__jki_lib_state_machine.vi"("State(s) in (\"\")"=w344) -> ("States Out"=w343:string)  [unwired: 14 in]
      }
      frame "Instruments: Init KH" {
        # "Reset KH7008 class"
        # "Template Separator\n(You can make a copy of, or modify, this frame)"
        n137 = Unbundle By Name(w359) -> ("C.E."=w354:refnum<class "Control Experiment.lvclass">)
        n138 = call "Insert Instrument Class by Name.vi"("error in (no error)"=w351, "Type"=T5 "KH7008", "Instrument in"=refnum<class "Instrument.lvclass"> refnum, "Control Experiment in"=w354) -> ("error out"=w352:errorcluster, "Control Experiment out"=w353:refnum<class "Control Experiment.lvclass">)  [unwired: 4 in, 2 out]
        n139 = for {
          tunnel: "KH Addresses" -> [w372] mode=indexing
          tunnel: w352 -> [w371]
          shift-right: [w369] -> w358
          shift-left: w353 -> [w370]
          tunnel: [w366] -> w357 mode=indexing
          tunnel: refnum<class "Instrument.KH7008.lvclass"> refnum ("element") -> [w365]
          n140 = call <userlib>:"Write Hardware Address.vi"("error in (no error)"=w371, "Address"=w372, "Instrument in"=w365) -> ("error out"=w368:errorcluster, "Instrument out"=w364:refnum<class "Instrument.KH7008.lvclass">)  [unwired: 7 in]
          n141 = call "Insert Instrument Class by Name.vi"("error in (no error)"=w368, "Type"=T5 "KH7008", "Instrument in"=w364, "Control Experiment in"=w370) -> ("error out"=w366:errorcluster, "Control Experiment out"=w369:refnum<class "Control Experiment.lvclass">)  [unwired: 4 in, 2 out]
        }
        n142 = Bundle By Name(cluster=w359, "C.E."=w358) -> (w360:T6)
        n143 = Merge Errors(w357) -> (w356:errorcluster)
        n144 = call <vilib>:"Add State(s) to Queue__jki_lib_state_machine.vi"("State(s) in (\"\")"=w363) -> ("States Out"=w362:string)  [unwired: 14 in]
      }
      frame "Instruments: Init Instruments" {
        # "Template Separator\n(You can make a copy of, or modify, this frame)"
        n145 = Unbundle By Name(w375) -> ("C.E."=w381:refnum<class "Control Experiment.lvclass">, "Installed Instruments"=w380:refnum<class "Instrument.lvclass">[], "Rings"=w382:refnum<vi>[])
        n146 = call <vilib>:"Get Cluster Information.vi"("error in (no error)"=w377, "variant"="Instruments (addresses)") -> ("error out"=w379:errorcluster, "cluster elements"=w383:variant[])  [unwired: 8 in]
        n147 = for {
          tunnel: w383 -> [w398] mode=indexing
          tunnel: w382 -> [w389] mode=indexing
          shift-right: [w395] -> w373
          shift-left: w381 -> [w396]
          tunnel: w379 -> [w394]
          tunnel: w380 -> [w391]
          tunnel: [w390] -> w374 mode=indexing
          n148 = property class="Ring"(reference=w389) -> ("RingText.Text"=w387:string, "Label.Text"=w392:string)  [unwired: 1 in, 2 out]
          n149 = Variant To Data(error in=w394, type="", Variant=w398) -> (data=w397:string, error out=w393:errorcluster)
          n150 = case shown="\"\"" w387 {
            selector: w387 -> [_ w408]
            tunnel: w397 -> [_ w416]
            tunnel: w396 -> [w404 w415]
            tunnel: [w403 w414] -> w395
            tunnel: w393 -> [w399 w407]
            tunnel: w392 -> [w401 w412]
            tunnel: w391 -> [_ w411]
            tunnel: [w400 w409] -> w390
            frame "" {
              n151 = call "Insert Instrument Class by Name.vi"("error in (no error)"=w399, "Type"=w401, "Instrument in"=refnum<class "Instrument.lvclass"> refnum, "Control Experiment in"=w404) -> ("error out"=w400:errorcluster, "Control Experiment out"=w403:refnum<class "Control Experiment.lvclass">)  [unwired: 4 in, 2 out]
            }
            frame Default {
              n152 = call "Find Class by Name.vi"("error in (no error)"=w407, "Name"=w408, "Installed Instruments"=w411) -> ("error out"=w406:errorcluster, "Instrument out"=w410:refnum<class "Instrument.lvclass">)  [unwired: 7 in]
              n153 = call <userlib>:"Write Hardware Address.vi"("error in (no error)"=w406, "Address"=w416, "Instrument in"=w410) -> ("error out"=w413:errorcluster, "Instrument out"=w405:refnum<class "Instrument.lvclass">)  [unwired: 7 in]
              n154 = call "Insert Instrument Class by Name.vi"("error in (no error)"=w413, "Type"=w412, "Instrument in"=w405, "Control Experiment in"=w415) -> ("error out"=w409:errorcluster, "Control Experiment out"=w414:refnum<class "Control Experiment.lvclass">)  [unwired: 4 in, 2 out]
            }
          }
        }
        n155 = Bundle By Name(cluster=w375, "C.E."=w373) -> (w376:T6)
        n156 = Merge Errors(w374) -> (w378:errorcluster)
        n157 = call <vilib>:"Add State(s) to Queue__jki_lib_state_machine.vi"("State(s) in (\"\")"=w386) -> ("States Out"=w385:string)  [unwired: 14 in]
      }
    }
  }
  n158 = Unbundle By Name(w6) -> ("C.E."=w4:refnum<class "Control Experiment.lvclass">)
  n159 = call "Control Experiment Class to JSON.vi"("error in (no error)"=w2, "Control Experiment in"=w4) -> ("error out"=→"error out":errorcluster, "Control Experiment out"=→"Control Experiment":refnum<class "Control Experiment.lvclass">)  [unwired: 7 in, 1 out]
